vi "Get Enable Debugging.vi"(8 "error in (no error)":errorcluster, 11 "NI_AB_API_Targetfile in":refnum<class "NI_AB_API_Targetfile.lvclass">) -> (0 "error out":errorcluster, 1 "Wait for debugger on launch":bool, 2 "Enable debugging":bool, 3 "NI_AB_API_Targetfile out":refnum<class "NI_AB_API_Targetfile.lvclass">)   [LabVIEW 2020, in "NI_AB_API_Targetfile.lvclass"]
uses:
  <vilib>/AppBuilder/AB_API/Targetfile/NI_AB_API_Targetfile.lvclass
  e:/builds/penguin/labview/branches/2020/dev/dist/vi.lib/AppBuilder/AB_API/Build/NI_AB_API_Build.lvclass
  <vilib>/AppBuilder/AB_Classes/TargetFile/AB_Targetfile.lvclass
  <vilib>/AppBuilder/AB_API/Targetfile/NI_AB_API_Targetfile.lvclass/NI_AB_API_Targetfile.ctl
  <vilib>/AppBuilder/AB_API/Build/NI_AB_API_Build.lvclass
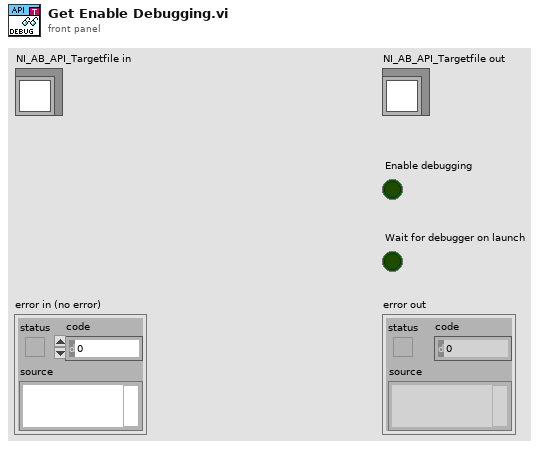
[diagram p1: front panel]
types:
  T1 = typedef "AB_Targetfile.ctl" = cluster{"targetfileName":string, "targetfileGUID":string, "enableDebugging":bool, "versionInfo":cluster{"productName":string, "legalCopyright":string, "companyName":string, "internalName":string, "fileDescription":string}, "eng_consolidatedTypeInfo":string, "fastFileFormat":bool, "eng_LEIFBuildData":u32, "versionIndependent":bool}
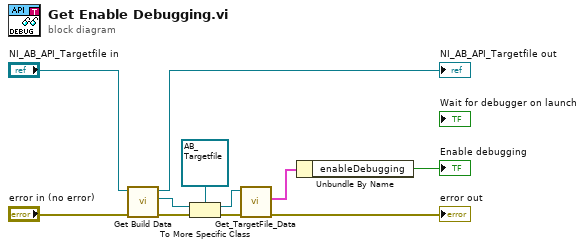
[diagram p0: block diagram]
diagram:
  n1 = call <vilib>:"Get Build Data.vi"("error in (no error)"="error in (no error)", "NI_AB_API_Build in"="NI_AB_API_Targetfile in") -> ("error out"=w3:errorcluster, "AB_Build.lvclass"=w5:refnum<class "AB_Build.lvclass">, "NI_AB_API_Build out"=→"NI_AB_API_Targetfile out":refnum<class "NI_AB_API_Targetfile.lvclass">)  [unwired: 7 in]
  n2 = To More Specific Class(target class=refnum<class "AB_Targetfile.lvclass"> refnum ("AB_Targetfile in"), reference=w5, error in=w3) -> (specific class reference=w4:refnum<class "AB_Targetfile.lvclass">, error out=w2:errorcluster)
  n3 = call <vilib>:"Get_TargetFile_Data.vi"("error in (no error)"=w2, "AB_Targetfile in"=w4) -> ("error out"=→"error out":errorcluster, "data"=w8:T1)  [unwired: 7 in, 1 out]
  n4 = Unbundle By Name(w8) -> ("enableDebugging"=→"Enable debugging":bool)
